vi "Get SBlock Type.vi"(8 "error in (no error)":errorcluster, 11 "Schedule Block in":refnum<class "Schedule Block.lvclass">) -> (0 "error out":errorcluster, 2 "SBlock Type":string, 3 "Schedule Block out":refnum<class "Schedule Block.lvclass">)   [LabVIEW 2020, in "Run Utilities.lvlib" / "Schedule Block.lvclass"]
doc: "Get the type of the SBlock based on the class name.\nThere are three types:\n- Non specific\n- Scan\n- Optimiser"
uses:
  Schedule Block.lvclass
  Schedule Block.lvclass/Schedule Block.ctl
  TALOS/TALOS_PPL.lvlibp
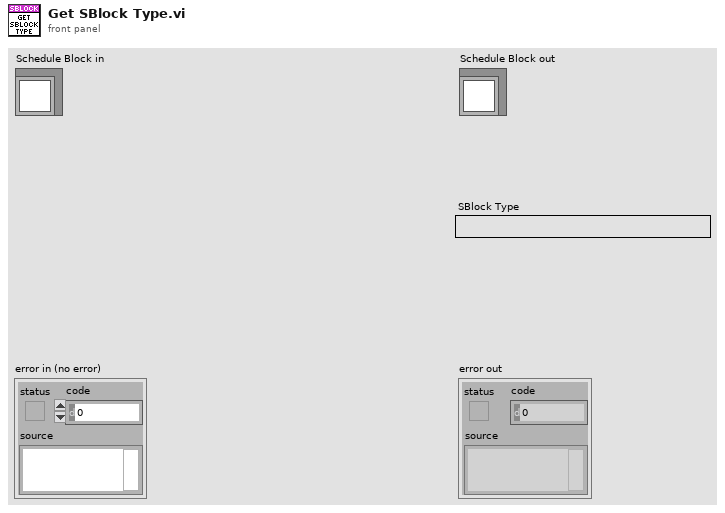
[diagram p1: front panel]
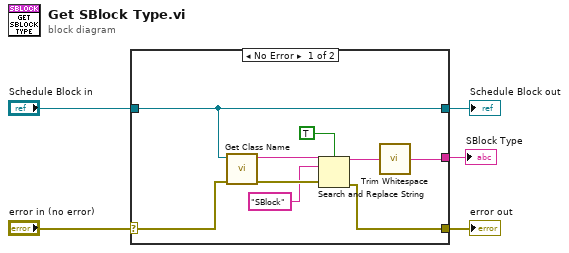
[diagram p0: block diagram]
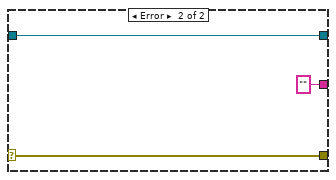
[diagram p2: hidden frame]
diagram:
  n1 = case shown="No Error" "error in (no error)" {
    selector: "error in (no error)" -> [w14 w17]
    tunnel: [w8 w17] -> w4
    tunnel: [w13 w16] -> w2
    tunnel: "Schedule Block in" -> [w13 w16]
    tunnel: [w6 "" ("Class Name")] -> w1
    frame No Error {
      n2 = call "Get Class Name.vi"("error in (no error)"=w14, "object"=w13) -> ("error out"=w9:errorcluster, "Class Name"=w12:string)  [unwired: 8 in]
      n3 = Search and Replace String(case sensitive?=TRUE ("ignore case? (F)"), input string=w12, search string="SBlock", error in=w9) -> (result string=w11:string, error out=w8:errorcluster)  [unwired: 4 in, 2 out]
      n4 = call <vilib>:"Trim Whitespace.vi"("string"=w11) -> ("trimmed string"=w6:string)  [unwired: 1 in]
    }
    frame Error {
    }
  }
  "error out" <- w4
  "Schedule Block out" <- w2
  "SBlock Type" <- w1
